vi "EVT Force IP.vi"(7 "defaultGateway":string, 9 "subnetMask":string, 10 "ipAddress":string, 11 "camera":u64) -> (3 "function return":u32(ring))   [LabVIEW 2019, in "EmergentCameraC.lvlib"]
doc: "EMERGENTCAMERAC_API EVT_ERROR EVT_ForceIP(Camera_Handle camera, const char* ipAddress, const char* subnetMask, const char* defaultGateway);"
uses:
  EmergentCameraC.lvlib
  emergentInstall_Windows/win64/eSDK/bin/EmergentCameraC.dll
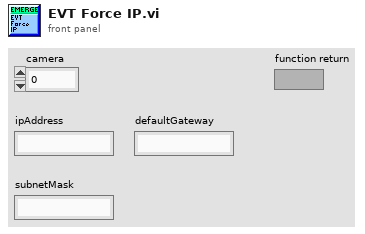
[diagram p1: front panel]
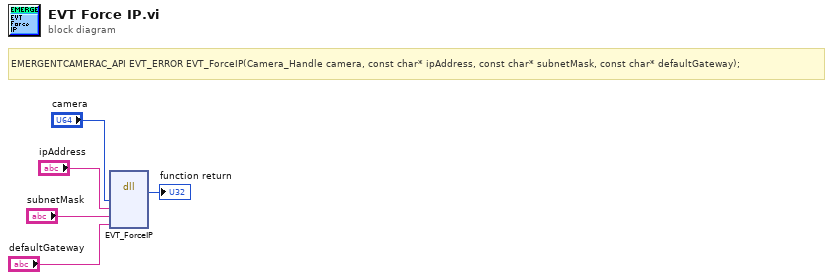
[diagram p0: block diagram]
diagram:
  # "EMERGENTCAMERAC_API EVT_ERROR EVT_ForceIP(Camera_Handle camera, const char* ipAddress, const char* subnetMask, const char* defaultGateway);"
  n1 = dll-call lib="E:/emergent/host-new_QT/emergentInstall_Windows/win64/eSDK/bin/EmergentCameraC.*" fn="EVT_ForceIP"("camera"="camera", "ipAddress"="ipAddress", "subnetMask"="subnetMask", "defaultGateway"="defaultGateway") -> (→"function return":u32)  [unwired: 7 in, 2 out]
